vi "TDMS Advanced Synchronous Write Speed Test.vi"() -> ()   [LabVIEW 2023]
doc: "This example demonstrates how to benchmark the streaming performance when you use the TDMS Advanced Synchronous Write function to write data to a .tdms file. This VI measures the time it takes to continuously write data from system memory to a .tdms file on the hard disk or a RAID array. This VI then calculates the average data throughput in bytes/second."
uses:
  <vilib>/Utility/tdmsutil.llb/TDMS Generate Random Data (I16).vi
panel:
  in  "Disable Buffering? (T)":bool=TRUE
  out "Bytes/second":dbl format="%#_4p"
  out "Current Number of Writes":i32
  out "Total Number of Writes":u64
  in  "Total Bytes to Write":u64=419430400
  in  "Write Block Size (bytes)":u64=4194304 step=1048576
  # "Overview: Demonstrates how to benchmark the streaming performance when you use the TDMS Advanced Synchronous Write function to write data to a .tdms file.\nInstructions:\nRun the VI. The file is created at [LabVIEW Data]\\Example TDMS Synchronous Speed Test Data.tdms."
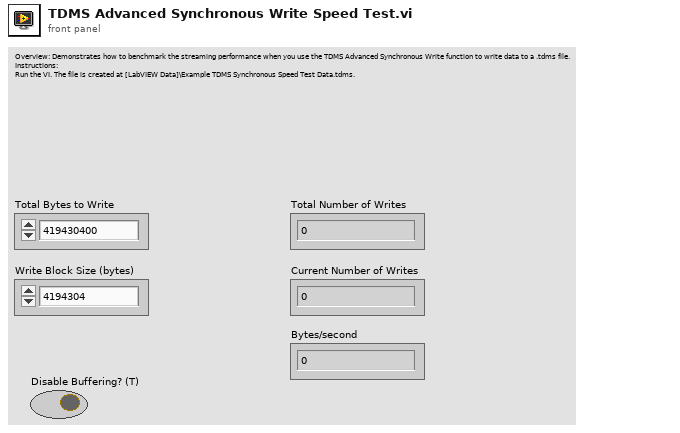
[diagram p1: front panel]
types:
  T1 = enum16{"open", "open or create", "create or replace", "create", "open (read-only)"}
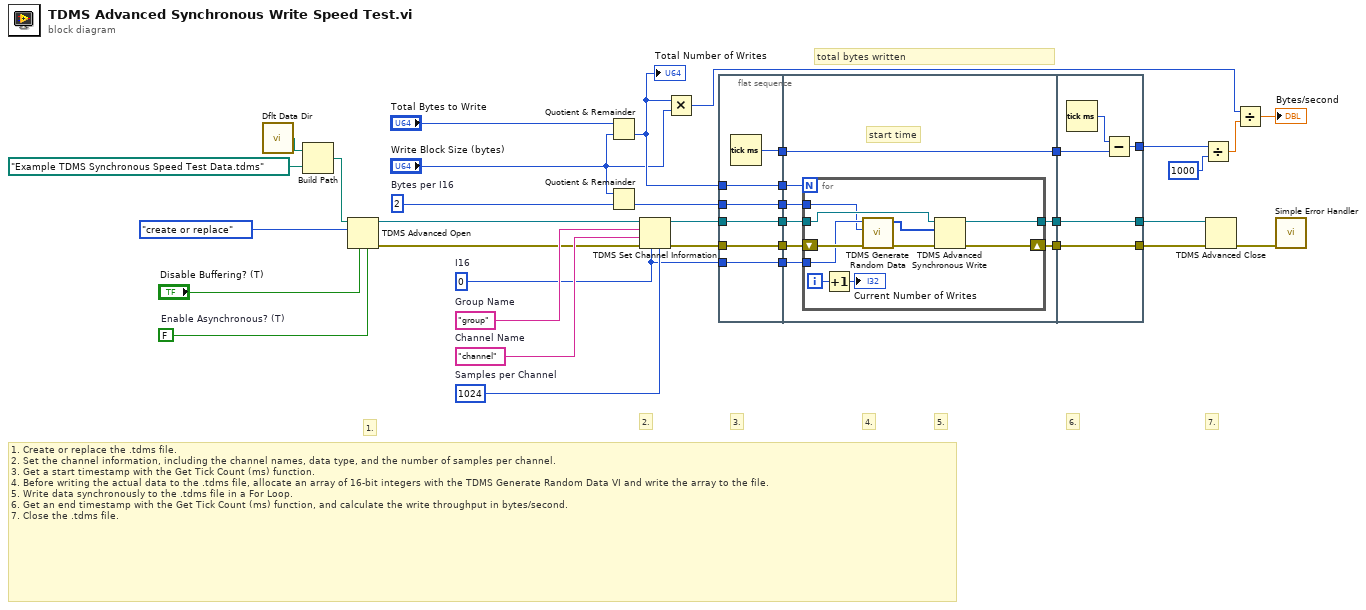
[diagram p0: block diagram]
diagram:
  w19 = FALSE  # Enable Asynchronous? (T)
  w23 = "group"  # Group Name
  w21 = u64 2  # Bytes per I16
  w25 = "channel"  # Channel Name
  w12 = i16 0  # I16
  w26 = u32 1024  # Samples per Channel
  # "total bytes written"
  # "7."
  # "4."
  # "6."
  # "5."
  # "3."
  # "2."
  # "1."
  # "1. Create or replace the .tdms file.  \n2. Set the channel information, including the channel names, data type, and the number of samples per channel.\n3. Get a start timestamp with the Get Tick Count (ms) function.\n4. Before writing the actual data to the .tdms file, allocate an array of 16-bit integers with the TDMS Generate Random Data VI and write the array to the file.\n5. Write data synchronously to the .tdms file in a For Loop. \n6. Get an end timestamp with the Get Tick Count (ms) function, and calculate the write throughput in bytes/second.\n7. Close the .tdms file."
  n1 = call <vilib>:"Dflt Data Dir.vi"() -> ("App:Default Data Directory"=w1:path)
  n2 = Build Path(base path=w1, name or relative path=path "Example TDMS Synchronous Speed Test Data.tdms") -> (appended path=w2:path)
  n3 = TDMS Advanced Open(4:w19, 6:"Disable Buffering? (T)", 10:T1."create or replace" ("operation (0:open)"), 11:w2) -> (0:w17:errorcluster, 3:w18:refnum<k34>)  [unwired: 1 in, 1 out]
  n4 = Quotient & Remainder(x="Total Bytes to Write", y="Write Block Size (bytes)") -> (floor(x/y)=w27:u64)  [unwired: 1 out]
  "Total Number of Writes" <- w27
  n5 = Quotient & Remainder(x="Write Block Size (bytes)", y=w21) -> (floor(x/y)=w10:u64)  [unwired: 1 out]
  n6 = TDMS Set Channel Information(4:w26, 6:w12, 8:w17, 9:w25, 10:w23, 11:w18) -> (0:w14:errorcluster, 3:w16:refnum<k34>)  [unwired: 1 in]
  n7 = Multiply(x=w27, y="Write Block Size (bytes)") -> (x*y=w5:u64)
  n8 = flat-sequence {
    tunnel: w16 -> [w42]
    tunnel: [w42] -> w36
    tunnel: [w41] -> w35
    tunnel: w27 -> [w40]
    tunnel: [w40] -> w34
    tunnel: [w39] -> w15
    tunnel: w14 -> [w39]
    tunnel: [w38] -> w13
    tunnel: w12 -> [w38]
    tunnel: [w37] -> w11
    tunnel: w10 -> [w37]
    tunnel: w36 -> [w50]
    tunnel: w35 -> [w49]
    tunnel: [w49] -> w33
    tunnel: [w48] -> w32
    tunnel: [w47] -> w31
    tunnel: w34 -> [w46]
    tunnel: w15 -> [w45]
    tunnel: w13 -> [w44]
    tunnel: w11 -> [w43]
    tunnel: w33 -> [w64]
    tunnel: w32 -> [w63]
    tunnel: [w63] -> w29
    tunnel: [w62] -> w28
    tunnel: w31 -> [w62]
    tunnel: [w61] -> w7
    frame #0 {
      n9 = Tick Count (ms)() -> (millisecond timer value=w41:u32)
    }
    frame #1 {
      # "start time"
      n10 = for {
        N: w46 -> [_]
        tunnel: [w57] -> w48
        shift-right: [w60] -> w47
        shift-left: w45 -> [w56]
        tunnel: w50 -> [w53]
        tunnel: w44 -> [w52]
        tunnel: w43 -> [w51]
        i -> [w59]
        n11 = Increment(x=w59) -> (x+1=→"Current Number of Writes":i32)
        n12 = call-poly <vilib>:"TDMS Generate Random Data.vi"("error in (no error)"=w56, "number of samples"=w51, "data type"=w52) -> ("error out"=w55:errorcluster, "data"=w54:i16[])  [unwired: 7 in]
        n13 = TDMS Advanced Synchronous Write(8:w55, 10:w54, 11:w53) -> (0:w60:errorcluster, 3:w57:refnum<k34>)
      }
    }
    frame #2 {
      n14 = Tick Count (ms)() -> (millisecond timer value=w65:u32)
      n15 = Subtract(x=w65, y=w64) -> (x-y=w61:u32)
    }
  }
  n16 = Divide(x=w7, y=u32 1000) -> (x/y=w8:dbl)
  n17 = TDMS Advanced Close(8:w28, 11:w29) -> (0:w30:errorcluster)  [unwired: 2 in, 1 out]
  n18 = Divide(x=w5, y=w8) -> (x/y=→"Bytes/second":dbl)
  n19 = call <vilib>:"Simple Error Handler.vi"("error in (no error)"=w30) -> ()  [unwired: 1 in, 8 out]
